vi "S2C_PCIe7841_Proc_SendLocalCmd.vi"(8 "Error In":errorcluster, 9 "ExeRef":refnum<vi>, 11 "Q-Ref":refnum<queue>) -> (0 "Error Out":errorcluster, 3 "Command":string)   [LabVIEW 2015]
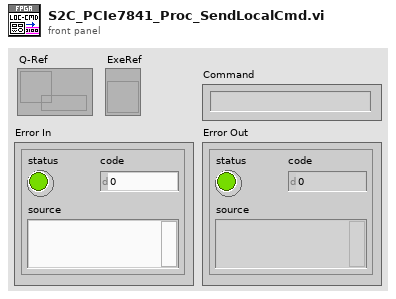
[diagram p1: front panel]
types:
  T1 = cluster{"Caller-Q":refnum<queue>, "Command":string, "Return":string, "Data":variant, "Timeout":dbl}
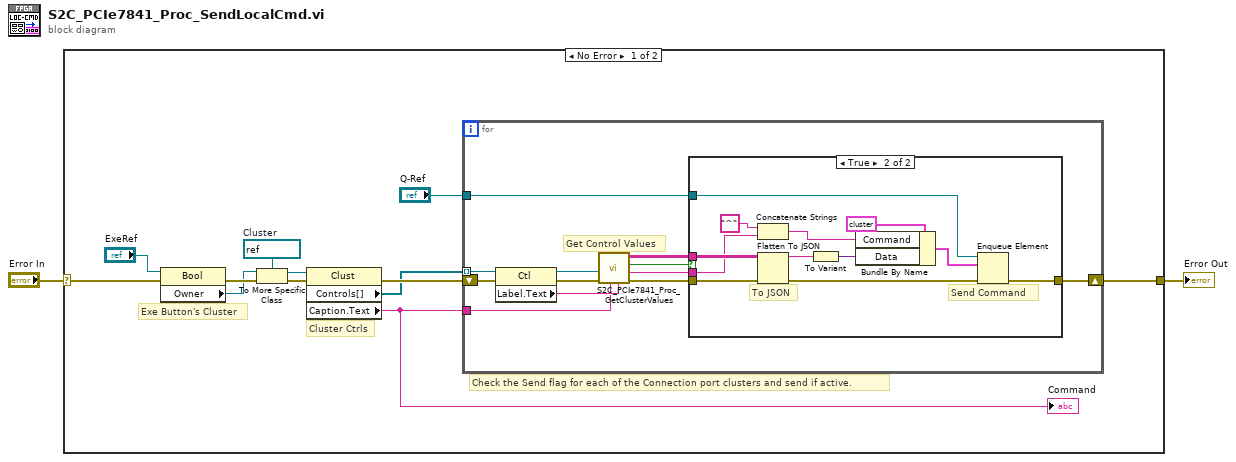
[diagram p0: block diagram]
diagram:
  n1 = case shown="No Error" "Error In" {
    selector: "Error In" -> [w13 w40]
    tunnel: [w4 w40] -> w1
    frame No Error {
      w10 = refnum<vi> refnum  # Cluster
      # "Check the Send flag for each of the Connection port clusters and send if active."
      # "Cluster Ctrls"
      # "Exe Button's Cluster"
      n2 = property class="Bool"(reference="ExeRef", error in=w13) -> (error out=w12:errorcluster, "Owner"=w11:refnum<vi>)  [unwired: 1 out]
      n3 = To More Specific Class(target class=w10, reference=w11, error in=w12) -> (specific class reference=w8:refnum<vi>, error out=w9:errorcluster)
      n4 = property class="Clust"(reference=w8, error in=w9) -> (error out=w7:errorcluster, "Controls[]"=w3:refnum<vi>[], "Caption.Text"=w6:string)  [unwired: 1 out]
      "Command" <- w6
      n5 = for {
        tunnel: w3 -> [w22] mode=indexing
        tunnel: w6 -> [w19]
        shift-right: [w18] -> w4
        shift-left: w7 -> [w26]
        tunnel: "Q-Ref" -> [w17]
        # "Get Control Values"
        n6 = property class="Ctl"(reference=w22, error in=w26) -> (reference out=w24:refnum<vi>, error out=w25:errorcluster, "Label.Text"=w23:string)
        n7 = call "S2C_PCIe7841_Proc_GetClusterValues.vi"("LabelText"=w23, "Cmd In"=w19, "Error In"=w25, "CtrlRef"=w24) -> ("Error Out"=w21:errorcluster, "Cmd Out"=w15:string, "Send?"=w16:bool, "Settings"=w20:string[][])  [unwired: 4 in]
        n8 = case shown="True" w16 {
          tunnel: w21 -> [w27 w32]
          tunnel: w20 -> [_ w31]
          tunnel: [w27 w30] -> w18
          tunnel: w17 -> [_ w29]
          tunnel: w15 -> [_ w28]
          frame False {
          }
          frame True {
            # "Send Command"
            # "To JSON"
            n9 = Concatenate Strings("^" ("string"), w28) -> (w36:string)
            n10 = Flatten To JSON(anything=w31, error in (no error)=w32) -> (JSON string=w34:string, 11:w33:errorcluster)  [unwired: 1 in]
            n11 = To Variant(anything=w34) -> (Variant=w38:variant)
            n12 = Bundle By Name(cluster=T1 {"Caller-Q"=refnum, "Command"="", "Return"="None", "Data"=variant, "Timeout"=10.0} ("element"), "Command"=w36, "Data"=w38) -> (w39:T1)
            n13 = Enqueue Element(queue=w29, element=w39, error in (no error)=w33) -> (error out=w30:errorcluster)  [unwired: 1 in, 2 out]
          }
        }
      }
    }
    frame Error {
    }
  }
  "Error Out" <- w1
